vi "panel1.vi"(8 "error in (no error)":errorcluster) -> (0 "error out":errorcluster)   [LabVIEW 2014]
uses:
  TagDB/_Support/Access/_variant.vi
  TagDB/_Support/Error/_[error50001]Can't Found Value.vi
  TagDB/_Support/Access/_setAnything.vi
  TagDB/_Support/Properties/tagDB dbChanged.vi
  TagDB/_Support/Private/_Cast TagDB Ref to DVR.vi
  TagDB/_global/URL/TRIM-BOTH-SPACE.vi
  TagDB/_Support/Error/_[error50000]Invalid DB REF.vi
  TagDB/_Support/Error/_[error50002]Invalid DataType.vi
  TagDB/_XNode/tagDB_setValue.xnode/tagDB_setValue.xnode
  TagDB/tagDB_Def.ctl
  TagDB/_XNode/tagDB_value.xnode/tagDB_value.xnode
  TagDB/TagDB(dev).lvlib
panel:
  in  "abcdef":T1={"number"=0, "boolean"=TRUE, "abcdef"={"number"=0, "boolean"=TRUE}}
  in  "value":string="test send message"
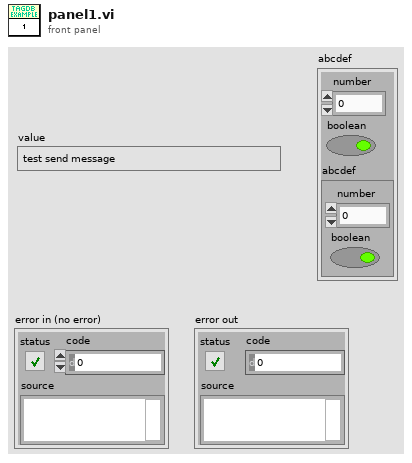
[diagram p1: front panel]
types:
  T1 = cluster{"number":i32, "boolean":bool, "abcdef":cluster{"number":i32, "boolean":bool}}
  T2 = typedef "TagDB(dev).lvlib/tagDB_Def.ctl" = refnum<k1>
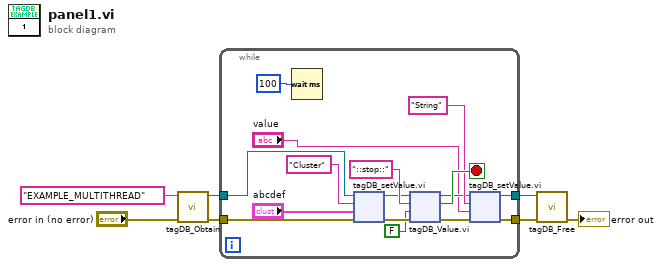
[diagram p0: block diagram]
diagram:
  n1 = call "tagDB_Obtain.vi"("error in (no error)"="error in (no error)", "name (unnamed)"="EXAMPLE_MULTITHREAD") -> ("error out"=w5:errorcluster, "DB"=w4:T2)  [unwired: 3 in, 1 out]
  n2 = while {
    tunnel: w4 -> [w12]
    tunnel: w5 -> [w10]
    tunnel: [w16] -> w7
    tunnel: [w19] -> w1
    stop <- w21 stop-if-true
    n3 = Wait (ms)(milliseconds to wait=u32 100) -> ()  [unwired: 1 out]
    n4 = xnode "tagDB_setValue.vi"("DB Ref"=w12, "name"="Cluster", "value"="abcdef", "Error In"=w10) -> ("DB Ref(dup)"=w11:T2, "Error Out"=w9:errorcluster)  [unwired: 1 out]
    n5 = xnode "tagDB_Value.vi"("error in (no error)"=w9, "DB Ref"=w11, "Type"=FALSE, "name"="::stop::") -> ("error out"=w18:errorcluster, "DB Ref(dup)"=w17:T2, "value"=w21:bool)  [unwired: 1 in]
    n6 = xnode "tagDB_setValue.vi"("DB Ref"=w17, "name"="String", "value"="value", "Error In"=w18) -> ("DB Ref(dup)"=w19:T2, "Error Out"=w16:errorcluster)  [unwired: 1 out]
  }
  n7 = call "tagDB_Free.vi"("error in (no error)"=w7, "DB Ref"=w1) -> ("error out"=→"error out":errorcluster)  [unwired: 9 in]
